vi "Config.vi"() -> ()   [LabVIEW 2020]
uses:
  Global_Variable/Global.vi
  <vilib>/Utility/config.llb/NI_LVConfig.lvlib
panel:
  in  "振动判定范围":T1={"频率检测段1范围"={"单位"="Hz", "下限"=0.0, "上限"=100.0}, "频率检测段2范围"={"单位"="Hz", "下限"=100.0, "上限"=1000.0}, "频率检测段3范围"={"单位"="Hz", "下限"=1000.0, "上限"=2000.0}, "频率检测段4范围"={"单位"="Hz", "下限"=2000.0, "上限"=3000.0}, "频率检测段5范围"={"单位"="Hz", "下限"=3000.0, "上限"=10000.0}}
  in  "振动判定":T2={"频率检测段1振幅"={"单位"="dB", "下限"=0.0, "上限"=50.0}, "频率检测段2振幅"={"单位"="dB", "下限"=0.0, "上限"=40.0}, "频率检测段3振幅"={"单位"="dB", "下限"=0.0, "上限"=40.0}, "频率检测段4振幅"={"单位"="dB", "下限"=0.0, "上限"=40.0}, "频率检测段5振幅"={"单位"="dB", "下限"=0.0, "上限"=40.0}}
  in  "产品型号":string(combo)
  in  "删除":bool
  in  "确定":bool
  in  "添加":bool
  in  "退出":bool
  in  "更新":bool
  # "NVH噪声检测"
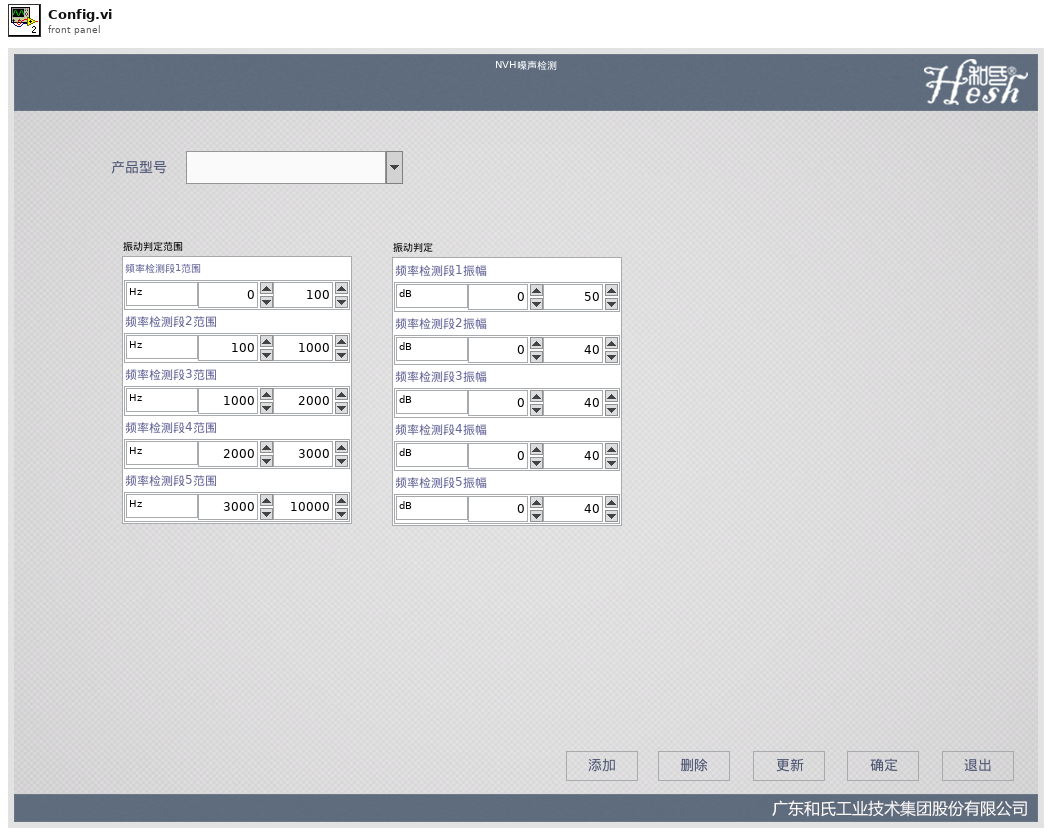
[diagram p1: front panel]
types:
  T1 = cluster{"频率检测段1范围":cluster{"单位":string, "下限":dbl, "上限":dbl}, "频率检测段2范围":cluster{"单位":string, "下限":dbl, "上限":dbl}, "频率检测段3范围":cluster{"单位":string, "下限":dbl, "上限":dbl}, "频率检测段4范围":cluster{"单位":string, "下限":dbl, "上限":dbl}, "频率检测段5范围":cluster{"单位":string, "下限":dbl, "上限":dbl}}
  T2 = cluster{"频率检测段1振幅":cluster{"单位":string, "下限":dbl, "上限":dbl}, "频率检测段2振幅":cluster{"单位":string, "下限":dbl, "上限":dbl}, "频率检测段3振幅":cluster{"单位":string, "下限":dbl, "上限":dbl}, "频率检测段4振幅":cluster{"单位":string, "下限":dbl, "上限":dbl}, "频率检测段5振幅":cluster{"单位":string, "下限":dbl, "上限":dbl}}
  T3 = typedef "NI_LVConfig.lvlib/Config Data RefNum.ctl" = refnum<k1>
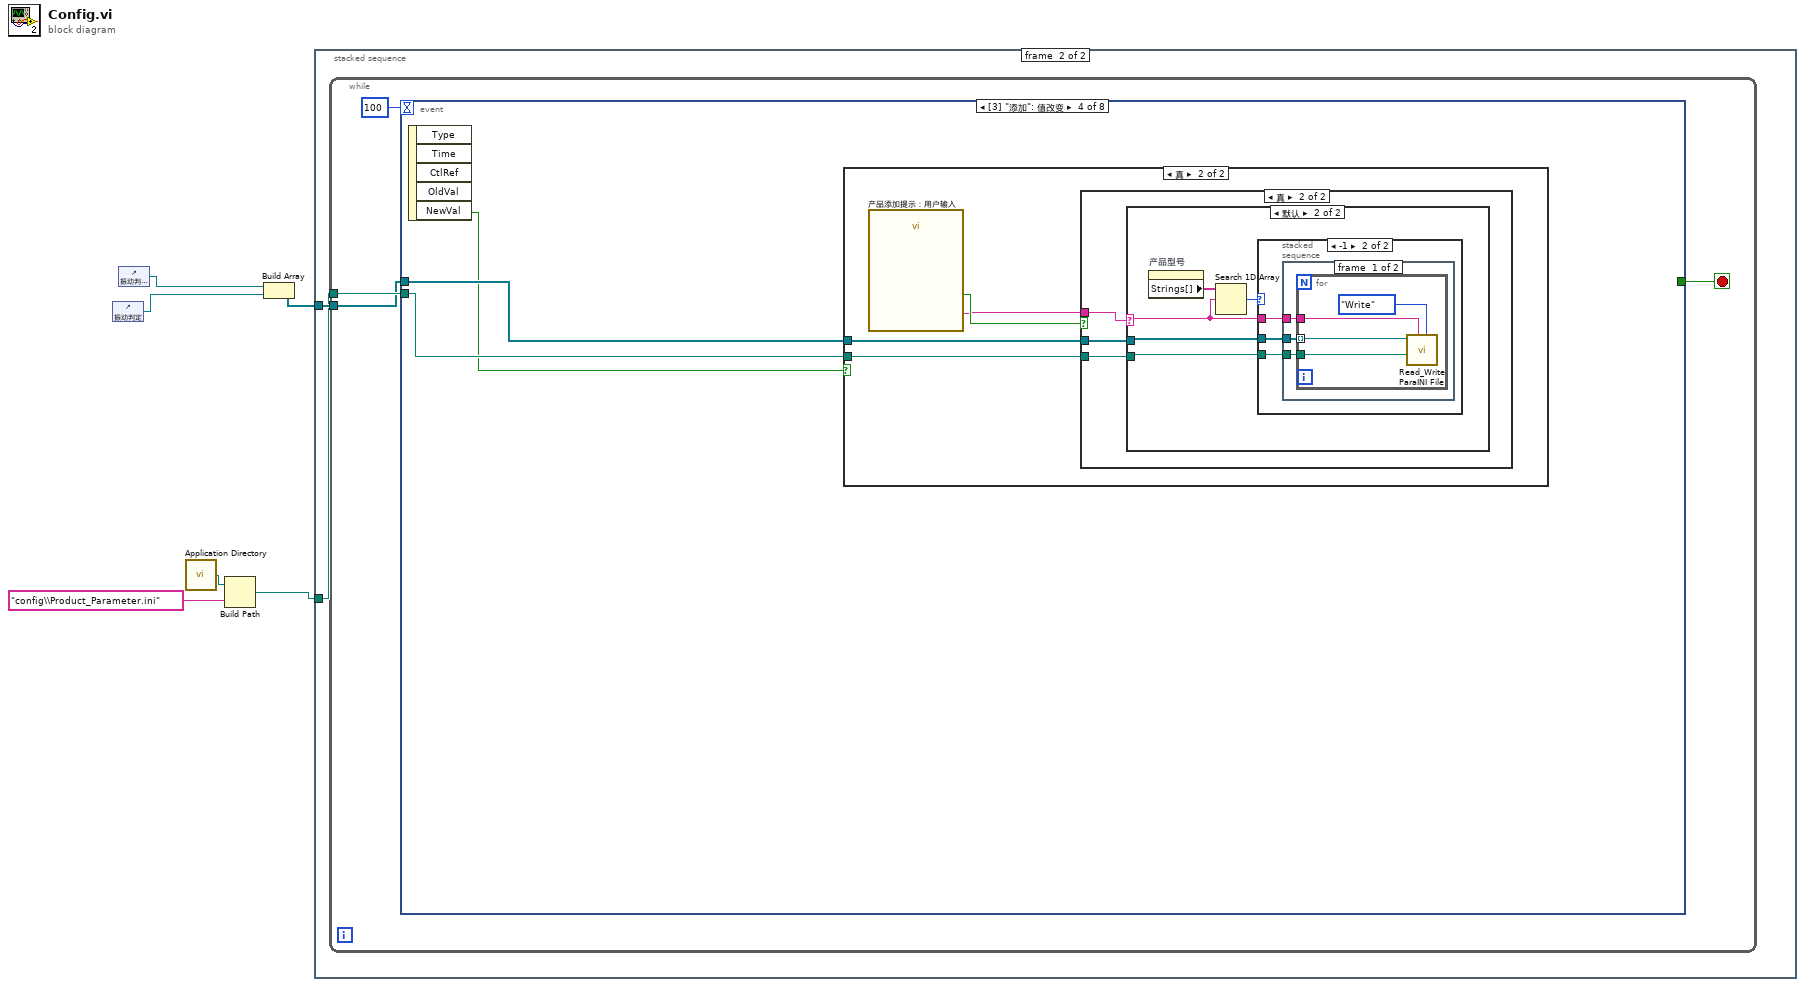
[diagram p0: block diagram]
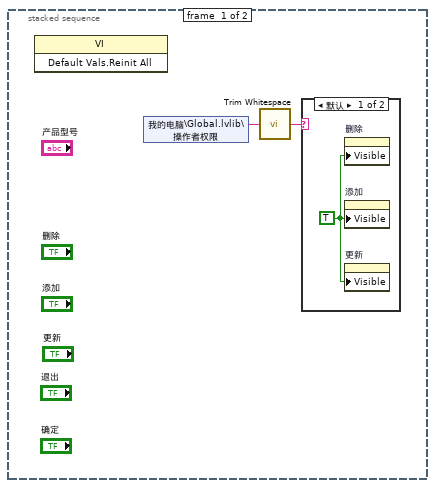
[diagram p2: hidden frame]
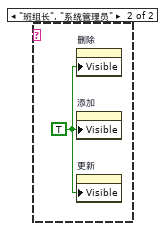
[diagram p3: hidden frame]
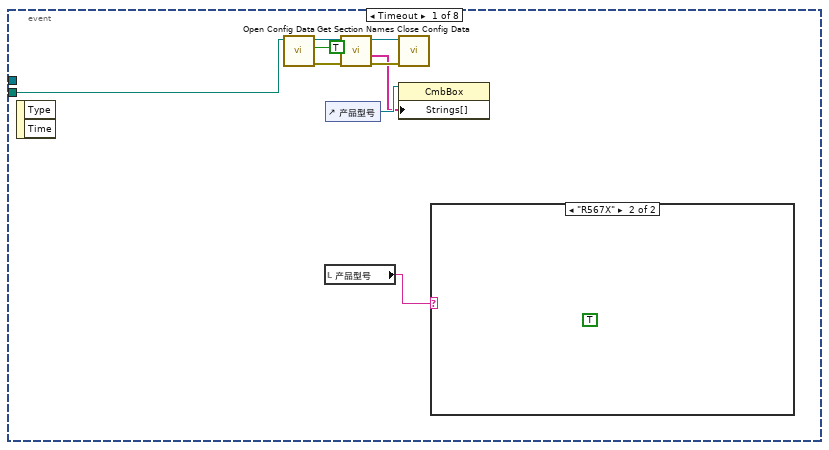
[diagram p4: hidden frame]
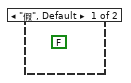
[diagram p5: hidden frame]
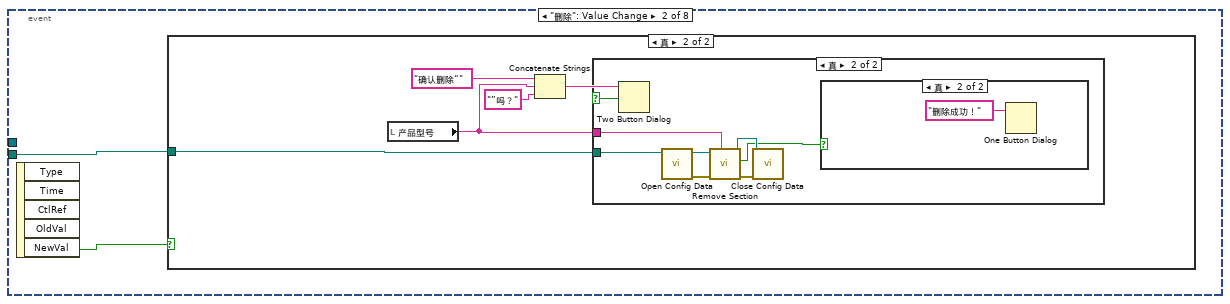
[diagram p6: hidden frame]
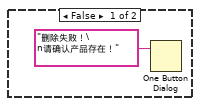
[diagram p9: hidden frame]
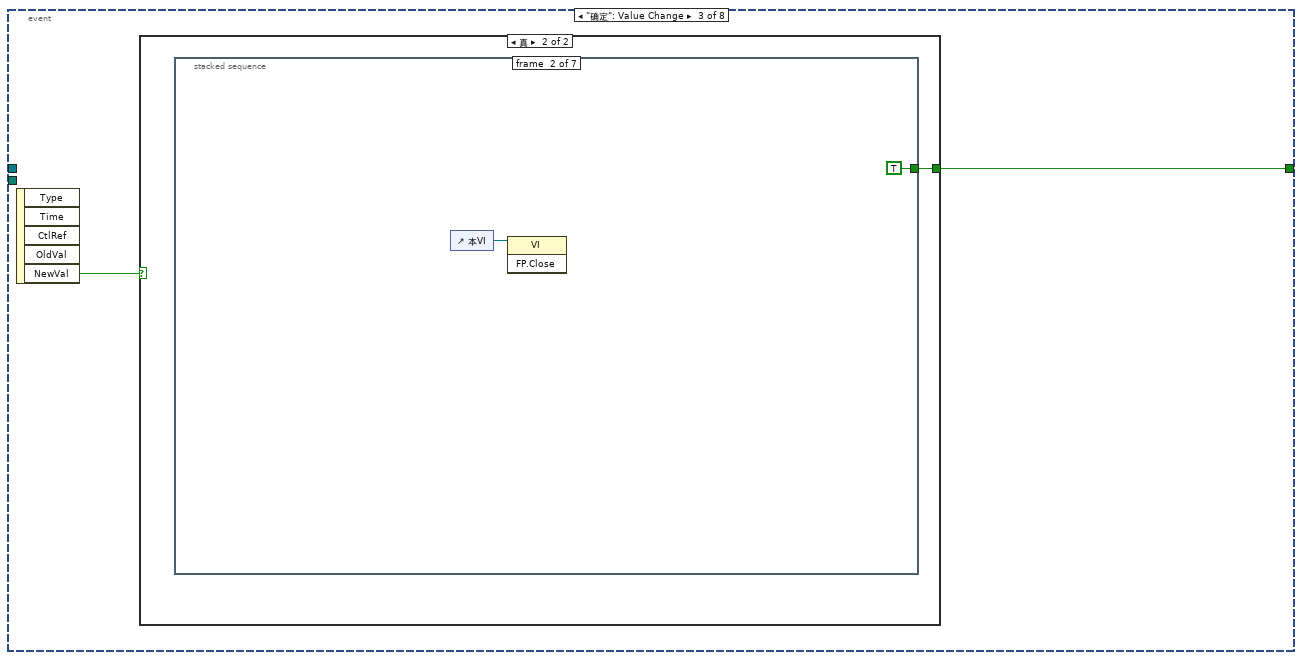
[diagram p10: hidden frame]
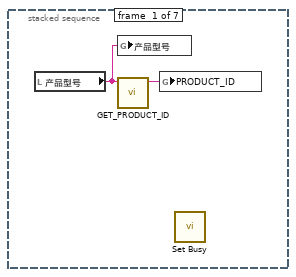
[diagram p12: hidden frame]
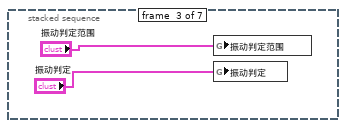
[diagram p13: hidden frame]
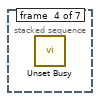
[diagram p14: hidden frame]
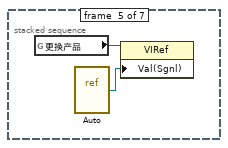
[diagram p15: hidden frame]
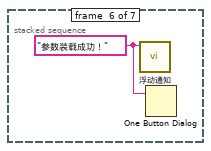
[diagram p16: hidden frame]
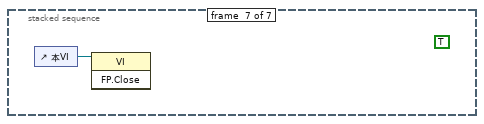
[diagram p17: hidden frame]
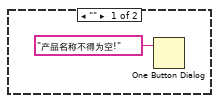
[diagram p20: hidden frame]
diagram:
  n1 = control-ref of="振动判定"() -> (w1:refnum<vi>)
  n2 = control-ref of="振动判定范围"() -> (w2:refnum<vi>)
  n3 = call <vilib>:"Application Directory.vi"() -> ("Application Directory"=w5:path)
  n4 = Build Path(base path=w5, name or relative path="config\\Product_Parameter.ini" ("名称或相对路径")) -> (appended path=w4:path)
  n5 = Build Array(w2, w1) -> (w6:refnum<vi>[])
  n6 = stacked-sequence {
    tunnel: w6 -> [_ w12]
    tunnel: w4 -> [_ w11]
    frame #0 {
      n7 = invoke class="VI" method="Default Vals.Reinit All"() -> ()  [unwired: 3 in, 3 out]
      n8 = shared-variable "我的电脑\\Global.lvlib\\操作者权限"() -> (w8:string)  [unwired: 1 in, 1 out]
      n9 = call <vilib>:"Trim Whitespace.vi"("string"=w8) -> ("trimmed string"=w7:string)  [unwired: 1 in]
      n10 = case shown="默认" w7 {
        frame Default {
          w9 = TRUE ("可见")
          n11 = property on="删除" class="Bool (严格)"("Visible"=w9) -> ()  [unwired: 2 in, 2 out]
          n12 = property on="添加" class="Bool (严格)"("Visible"=w9) -> ()  [unwired: 2 in, 2 out]
          n13 = property on="更新" class="Bool (严格)"("Visible"=w9) -> ()  [unwired: 2 in, 2 out]
        }
        frame "班组长", "系统管理员" {
          w10 = TRUE ("可见")
          n14 = property on="删除" class="Bool (严格)"("Visible"=w10) -> ()  [unwired: 2 in, 2 out]
          n15 = property on="添加" class="Bool (严格)"("Visible"=w10) -> ()  [unwired: 2 in, 2 out]
          n16 = property on="更新" class="Bool (严格)"("Visible"=w10) -> ()  [unwired: 2 in, 2 out]
        }
      }
    }
    frame #1 {
      n17 = while {
        tunnel: w11 -> [w16]
        tunnel: w12 -> [w14]
        stop <- w15 stop-if-true
        n18 = event shown="[3] \"添加\": 值改变" {
          selector: _ -> [_ _ _ _ _ _ _ _]
          dyn-events: _ -> [_ _ _ _ _ _ _ _]
          timeout: 100 -> [_ _ _ _ _ _ _ _]
          tunnel: w16 -> [w20 w27 _ w57 w85 _ w101 _]
          tunnel: [_ _ w43 _ _ TRUE _ TRUE] -> w15
          tunnel: w14 -> [_ _ _ w58 w86 _ w100 _]
          event Timeout {
            n19 = event-data() -> ()  [unwired: 1 in, 2 out]
            n20 = call <vilib>:"Open Config Data.vi"("create file if necessary (T)"=TRUE, "configuration file path"=w20) -> ("error out"=w22:errorcluster, "refnum"=w21:T3)  [unwired: 7 in, 1 out]
            n21 = local read "产品型号"() -> (w17:string)
            n22 = control-ref of="产品型号"() -> (w19:refnum<vi>)
            n23 = call <vilib>:"Get Section Names.vi"("error in (no error)"=w22, "refnum"=w21) -> ("error out"=w24:errorcluster, "section names"=w18:string[], "refnum out"=w23:T3)  [unwired: 7 in]
            n24 = call <vilib>:"Close Config Data.vi"("error in (no error)"=w24, "refnum"=w23) -> ()  [unwired: 8 in, 2 out]
            n25 = property on="属性节点" class="CmbBox"(reference=w19, "Strings[]"=w18) -> ()  [unwired: 1 in, 2 out]
            n26 = case shown="\"R567X\"" w17 {
              frame "假", Default {
                (unwired) FALSE ("可见")
              }
              frame "R567X" {
                (unwired) TRUE ("可见")
              }
            }
          }
          event "删除": Value Change {
            n27 = event-data() -> ("NewVal"=w26:bool)  [unwired: 1 in, 4 out]
            n28 = case shown="真" w26 {
              tunnel: w27 -> [_ w29]
              frame False {
              }
              frame True {
                n29 = local read "产品型号"() -> (w28:string)
                n30 = Concatenate Strings("确认删除“", w28, "”吗？") -> (w31:string)
                n31 = Two Button Dialog(message=w31) -> (T button?=w30:bool)  [unwired: 2 in]
                n32 = case shown="真" w30 {
                  tunnel: w29 -> [_ w35]
                  tunnel: w28 -> [_ w34]
                  frame False {
                  }
                  frame True {
                    n33 = call <vilib>:"Open Config Data.vi"("configuration file path"=w35) -> ("error out"=w37:errorcluster, "refnum"=w40:T3)  [unwired: 8 in, 1 out]
                    n34 = call <vilib>:"Remove Section.vi"("section"=w34, "error in (no error)"=w37, "refnum"=w40) -> ("error out"=w39:errorcluster, "section exists?"=w36:bool, "refnum out"=w38:T3)  [unwired: 6 in]
                    n35 = call <vilib>:"Close Config Data.vi"("error in (no error)"=w39, "refnum"=w38) -> ()  [unwired: 8 in, 2 out]
                    n36 = case shown="真" w36 {
                      frame False {
                        n37 = One Button Dialog(message="删除失败！\n请确认产品存在！" ("消息")) -> ()  [unwired: 1 in, 1 out]
                      }
                      frame True {
                        n38 = One Button Dialog(message="删除成功！" ("消息")) -> ()  [unwired: 1 in, 1 out]
                      }
                    }
                  }
                }
              }
            }
          }
          event "确定": Value Change {
            n39 = event-data() -> ("NewVal"=w44:bool)  [unwired: 1 in, 4 out]
            n40 = case shown="真" w44 {
              tunnel: [_ w45] -> w43
              frame False {
              }
              frame True {
                n41 = stacked-sequence {
                  tunnel: [_ TRUE _ _ _ _ _] -> w45
                  frame #0 {
                    n42 = local read "产品型号"() -> (w47:string)
                    n43 = global write "Global.vi" "产品型号"(w47) -> ()
                    n44 = call "GET_PRODUCT_ID.vi"("PRODFUCT_NAME"=w47) -> ("PRODUCT_ID"=w46:string)  [unwired: 10 in]
                    n45 = global write "追溯Global.vi" "PRODUCT_ID"(w46) -> ()
                    n46 = call <vilib>:"Set Busy.vi"() -> ()  [unwired: 10 in, 2 out]
                  }
                  frame #1 {
                    n47 = control-ref of="本VI"() -> (w49:refnum<vi>)
                    n48 = invoke class="VI" method="FP.Close"(reference=w49) -> ()  [unwired: 2 in, 3 out]
                  }
                  frame #2 {
                    n49 = global write "判定参数.vi" "振动判定范围"("振动判定范围") -> ()
                    n50 = global write "判定参数.vi" "振动判定"("振动判定") -> ()
                  }
                  frame #3 {
                    n51 = call <vilib>:"Unset Busy.vi"() -> ()  [unwired: 11 in, 1 out]
                  }
                  frame #4 {
                    n52 = global read "Global.vi" "更换产品"() -> (w53:refnum<vi>)
                    n53 = vi-ref "Auto.vi"() -> (w52:refnum<vi>)
                    n54 = property class="VIRef"(reference=w53, "Val(Sgnl)"=w52) -> ()  [unwired: 1 in, 2 out]
                  }
                  frame #5 {
                    w54 = "参数装载成功！" ("消息")
                    n55 = call "浮动通知.vi"("通知内容"=w54) -> ()  [unwired: 11 in]
                    n56 = One Button Dialog(message=w54) -> ()  [unwired: 1 in, 1 out]
                  }
                  frame #6 {
                    (unwired) TRUE
                    n57 = control-ref of="本VI"() -> (w55:refnum<vi>)
                    n58 = invoke class="VI" method="FP.Close"(reference=w55) -> ()  [unwired: 2 in, 3 out]
                  }
                }
              }
            }
          }
          event "添加": Value Change {
            n59 = event-data() -> ("NewVal"=w56:bool)  [unwired: 1 in, 4 out]
            n60 = case shown="真" w56 {
              tunnel: w58 -> [_ w62]
              tunnel: w57 -> [_ w61]
              frame False {
              }
              frame True {
                n61 = call "产品添加提示：用户输入"() -> ("产品型号"=w59:string, "确定"=w60:bool)  [unwired: 17 in, 1 out]
                n62 = case shown="真" w60 {
                  tunnel: w62 -> [_ w65]
                  tunnel: w61 -> [_ w64]
                  tunnel: w59 -> [_ w63]
                  frame False {
                  }
                  frame True {
                    n63 = case shown="默认" w63 {
                      selector: w63 -> [_ w68]
                      tunnel: w65 -> [_ w71]
                      tunnel: w64 -> [_ w70]
                      frame "" {
                        n64 = One Button Dialog(message="产品名称不得为空!" ("text")) -> ()  [unwired: 1 in, 1 out]
                      }
                      frame Default {
                        n65 = property on="产品型号" class="CmbBox"() -> ("Strings[]"=w69:string[])  [unwired: 2 in, 2 out]
                        n66 = Search 1D Array(1D array=w69, element=w68) -> (index of element=w67:i32)  [unwired: 1 in]
                        n67 = case shown="-1" w67 {
                          tunnel: w71 -> [_ w75]
                          tunnel: w70 -> [_ w74]
                          tunnel: w68 -> [_ w73]
                          frame Default {
                            n68 = One Button Dialog(message="产品已存在！" ("消息")) -> ()  [unwired: 1 in, 1 out]
                          }
                          frame -1 {
                            n69 = stacked-sequence {
                              tunnel: w75 -> [w78 _]
                              tunnel: w74 -> [w77 _]
                              tunnel: w73 -> [w76 _]
                              frame #0 {
                                n70 = for {
                                tunnel: w78 -> [w79] mode=indexing
                                tunnel: w77 -> [w81]
                                tunnel: w76 -> [w80]
                                n71 = call "Read_Write ParaINI File.vi"("Mode"=enum16{"Read", "Write"}."Write", "Section"=w80, "Filepath"=w81, "Ctl Refnum"=w79) -> ()  [unwired: 7 in, 1 out]
                                }
                              }
                              frame #1 {
                                n72 = One Button Dialog(message="添加成功！" ("消息")) -> ()  [unwired: 1 in, 1 out]
                              }
                            }
                          }
                        }
                      }
                    }
                  }
                }
              }
            }
          }
          event "产品型号": Value Change {
            n73 = event-data() -> ("NewVal"=w84:string)  [unwired: 1 in, 4 out]
            n74 = stacked-sequence {
              tunnel: w86 -> [_ _ w89]
              tunnel: w85 -> [_ _ w94]
              tunnel: w84 -> [_ w88 _]
              frame #0 {
                n75 = control-ref of="本VI"() -> (w87:refnum<vi>)
                n76 = invoke class="VI" method="Default Vals.Reinit All"(reference=w87) -> ()  [unwired: 2 in, 3 out]
              }
              frame #1 {
                n77 = local write "产品型号"(w88) -> ()
              }
              frame #2 {
                n78 = local read "产品型号"() -> (w93:string)
                n79 = call <vilib>:"Set Busy.vi"() -> ("error out"=w91:errorcluster)  [unwired: 10 in, 1 out]
                n80 = call "Read_Write INI File.vi"("Mode"=enum16{"Read", "Write"}."Read", "Section"=w93, "error in"=w91, "Filepath"=w94, "Ctl Refnum"=w89) -> ("error out"=w90:errorcluster)  [unwired: 6 in]
                n81 = call <vilib>:"Unset Busy.vi"("error in (no error)"=w90) -> ()  [unwired: 10 in, 1 out]
              }
            }
          }
          event "退出": Value Change {
            n82 = event-data() -> ()  [unwired: 1 in, 5 out]
            n83 = control-ref of="本VI"() -> (w97:refnum<vi>)
            n84 = invoke class="VI" method="FP.Close"(reference=w97) -> (reference out=w95:refnum<vi>, error out=w96:errorcluster)  [unwired: 2 in, 1 out]
            n85 = Close Reference(reference=w95, error in (no error)=w96) -> ()  [unwired: 1 out]
          }
          event "更新": Value Change {
            n86 = event-data() -> ("NewVal"=w99:bool)  [unwired: 1 in, 4 out]
            n87 = case shown="真" w99 {
              tunnel: w101 -> [_ w106]
              tunnel: w100 -> [_ w102]
              frame False {
              }
              frame True {
                n88 = local read "产品型号"() -> (w104:string)
                n89 = call "Read_Write INI File.vi"("Mode"=enum16{"Read", "Write"}."Write", "Section"=w104, "Filepath"=w106, "Ctl Refnum"=w102) -> ("error out"=w103:errorcluster)  [unwired: 7 in]
                n90 = case shown="无错误" w103 {
                  frame No Error {
                    n91 = Wait (ms)(milliseconds to wait=u32 500 ("等待时间（毫秒）")) -> ()  [unwired: 1 out]
                    n92 = One Button Dialog(message="更新成功！" ("通知内容")) -> ()  [unwired: 1 in, 1 out]
                  }
                  frame Error {
                    n93 = Wait (ms)(milliseconds to wait=u32 500 ("等待时间（毫秒）")) -> ()  [unwired: 1 out]
                    n94 = call "浮动通知.vi"("通知内容"="更新失败！") -> ()  [unwired: 11 in]
                  }
                }
              }
            }
          }
          event Panel Close {
            n95 = event-data() -> ()  [unwired: 1 in, 3 out]
          }
        }
      }
    }
  }
